vi "json Parse String Array - array path.vi"(8 "error in (no error)":errorcluster, 9 "default":string[](array[string]), 10 "path":string[](array[string]), 11 "JSON Document in":refnum<class "JSON Document.lvclass">) -> (0 "error out":errorcluster, 1 "defaulted?":bool, 2 "value":string[](array[string]), 3 "JSON Document out":refnum<class "JSON Document.lvclass">, 4 "elements defaulted?":bool[](array[boolean]))   [LabVIEW 2015, in "JSON Document.lvclass"]
uses:
  JSON Document.lvclass
  json Parse String Array - string path.vi
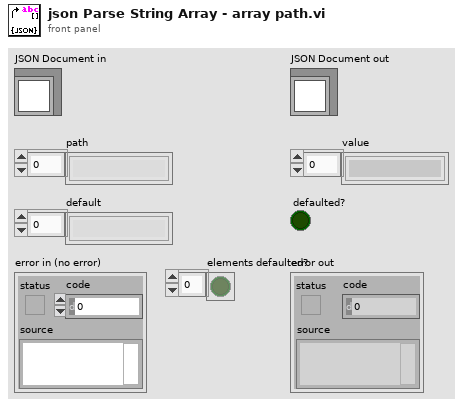
[diagram p1: front panel]
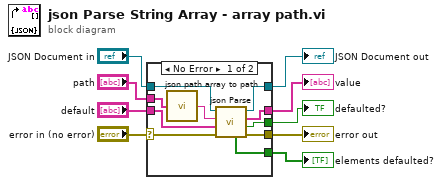
[diagram p0: block diagram]
diagram:
  n1 = case shown="No Error" "error in (no error)" {
    selector: "error in (no error)" -> [w14 w22]
    tunnel: [w15 w22] -> w8
    tunnel: [w17 w21] -> w6
    tunnel: "JSON Document in" -> [w18 w21]
    tunnel: "default" -> [w13 w20]
    tunnel: "path" -> [w10 _]
    tunnel: [w12 w20] -> w3
    tunnel: [w16 _] -> w2
    tunnel: [w11 _] -> w1
    frame No Error {
      n2 = call "json path array to path.vi"("path"=w10) -> ("String"=w19:string)
      n3 = call-poly "json Parse.vi"("error in (no error)"=w14, "default"=w13, "path"=w19, "JSON Document in"=w18) -> ("error out"=w15:errorcluster, "defaulted?"=w16:bool, "value"=w12:string[], "JSON Document out"=w17:refnum<class "JSON Document.lvclass">, "elements defaulted?"=w11:bool[])  [unwired: 3 in]
    }
    frame Error {
    }
  }
  "error out" <- w8
  "JSON Document out" <- w6
  "value" <- w3
  "defaulted?" <- w2
  "elements defaulted?" <- w1
